vi "Host cRIO Interface.vi"() -> ()   [LabVIEW 2017]
uses:
  <vilib>/FPGAPlugInAG/NI 9159/niLvFpga_Open_NI 9159.vi
  <vilib>/rvi/interface/common/dynamic/niFpgaDynamicAddResources.vi
  <vilib>/FPGAPlugInAG/Dynamic/niLvFpga_Run_Dynamic.vi
  <vilib>/Utility/error.llb/Error Cluster From Error Code.vi
  <vilib>/rvi/errors/niLvFpgaAdjustHostInterfaceError.vi
  <vilib>/FPGAPlugInAG/Dynamic/niLvFpga_Close_Dynamic.vi
  <vilib>/rvi/interface/nirviOpenFPGA/nirviOpenFPGA.xnode
  FPGA Bitfiles/RIOExpansionLate_FPGATarget2_9159FPGADMATop_ueHRLpdidM4.lvbitx
  <vilib>/rvi/interface/nirviMethod/nirviMethod.xnode
  <vilib>/rvi/interface/nirviCloseFPGA/nirviCloseFPGA.xnode
  <vilib>/FPGAPlugInAG/Dynamic/niLvFpga_ReadFifo_Dynamic.vi
  <vilib>/rvi/errors/niLvFpgaMergeErrorWithErrorCode.vi
panel:
  out "Lo":u32[](array[numeric])
  out "Hi":u32[](array[numeric])
  out "error out":errorcluster
  in  "stop":bool
  out "Elements Remaining":u32
  out "Data":u64[](array[numeric])
  in  "Number of Elements":u32
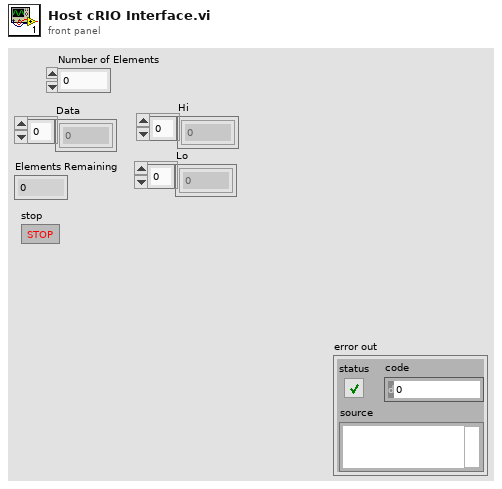
[diagram p1: front panel]
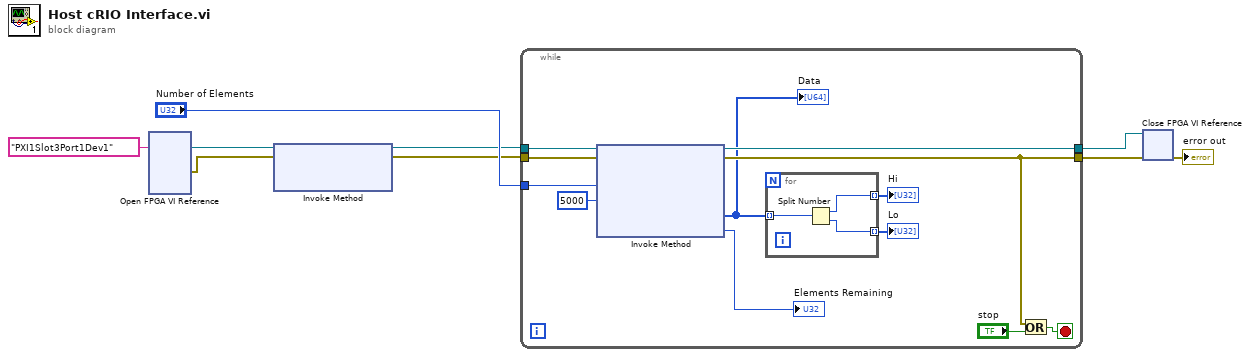
[diagram p0: block diagram]
diagram:
  n1 = xnode "Open FPGA VI Reference"("resource name"=tag "PXI1Slot3Port1Dev1") -> ("FPGA VI Reference Out"=w4:refnum<k20>, "error out"=w3:errorcluster)  [unwired: 1 in]
  n2 = xnode "Invoke Method"("FPGA VI Reference In"=w4, "error in"=w3) -> ("FPGA VI Reference Out"=w2:refnum<k20>, "error out"=w1:errorcluster)  [unwired: 1 in]
  n3 = while {
    tunnel: w2 -> [w21]
    tunnel: w1 -> [w20]
    tunnel: "Number of Elements" -> [w19]
    tunnel: [w15] -> w8
    tunnel: [w14] -> w7
    stop <- w13 stop-if-true
    n4 = xnode "Invoke Method"("FPGA VI Reference In"=w21, "error in"=w20, "Number of Elements"=w19, "Timeout (ms)"=5000) -> ("FPGA VI Reference Out"=w14:refnum<k20>, "error out"=w15:errorcluster, "Data"=w12:u64[], "Elements Remaining"=→"Elements Remaining":u32)
    "Data" <- w12
    n5 = for {
      tunnel: w12 -> [w24] mode=indexing
      tunnel: [w23] -> w11 mode=indexing
      tunnel: [w22] -> w10 mode=indexing
      n6 = Split Number(x=w24) -> (hi(x)=w23:u32, lo(x)=w22:u32)
    }
    "Hi" <- w11
    "Lo" <- w10
    n7 = Or(x=w15, y="stop") -> (x .or. y?=w13:bool)
  }
  n8 = xnode "Close FPGA VI Reference"("FPGA VI Reference In"=w7, "error in"=w8) -> ("error out"=→"error out":errorcluster)
